vi "JoystickControls.vi"() -> (3 "input cluster":T1)   [LabVIEW 2015]
uses:
  Controls.ctl
  References/Refnums.vi
  <vilib>/Rock Robotics/WPI/Utilities/WPI_GetSetVariantRefNum.vi
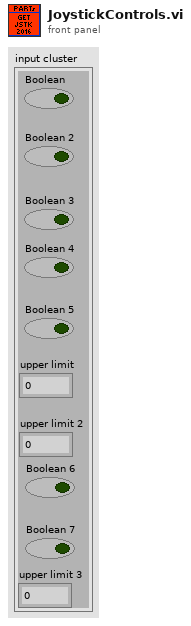
[diagram p1: front panel]
types:
  T1 = typedef "Controls.ctl" = cluster{"Boolean":bool, "Boolean 2":bool, "Boolean 3":bool, "Boolean 4":bool, "Boolean 5":bool, "upper limit":dbl, "upper limit 2":dbl, "Boolean 6":bool, "Boolean 7":bool, "upper limit 3":dbl}
  T2 = typedef "WPI_JoystickDevRef.ctl" = cluster{"Device":T3}
  T3 = typedef "WPI_JoystickDeviceEnum.ctl" = enum16{"USB 0", "USB 1", "USB 2", "USB 3", "USB 4", "USB 5"}
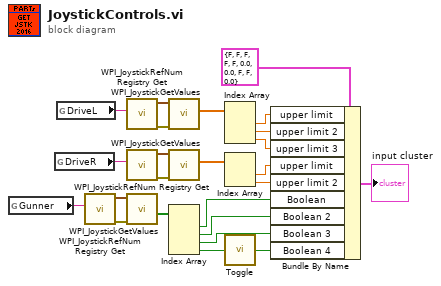
[diagram p0: block diagram]
diagram:
  n1 = global read "Refnums.vi" "Gunner"() -> (w23:string)
  n2 = global read "Refnums.vi" "DriveR"() -> (w8:string)
  n3 = global read "Refnums.vi" "DriveL"() -> (w22:string)
  n4 = call <vilib>:"WPI_JoystickRefNum Registry Get.vi"("refnum name"=w23) -> ("error out"=w18:errorcluster, "JoystickDevRef"=w19:T2)  [unwired: 9 in]
  n5 = call <vilib>:"WPI_JoystickRefNum Registry Get.vi"("refnum name"=w22) -> ("error out"=w21:errorcluster, "JoystickDevRef"=w20:T2)  [unwired: 9 in]
  n6 = call <vilib>:"WPI_JoystickRefNum Registry Get.vi"("refnum name"=w8) -> ("error out"=w9:errorcluster, "JoystickDevRef"=w10:T2)  [unwired: 9 in]
  n7 = call <vilib>:"WPI_JoystickGetValues.vi"("error in (no error)"=w18, "JoystickDevRef"=w19) -> ("Buttons"=w24:bool[])  [unwired: 5 in, 4 out]
  n8 = call <vilib>:"WPI_JoystickGetValues.vi"("error in (no error)"=w21, "JoystickDevRef"=w20) -> ("Axes"=w15:dbl[])  [unwired: 5 in, 4 out]
  n9 = call <vilib>:"WPI_JoystickGetValues.vi"("error in (no error)"=w9, "JoystickDevRef"=w10) -> ("Axes"=w11:dbl[])  [unwired: 5 in, 4 out]
  n10 = Index Array(array=w24) -> (element #1=w5:bool, element #2=w4:bool, element #3=w3:bool, element #4=w2:bool)  [unwired: 4 in]
  n11 = Index Array(array=w15) -> (element #1=w14:dbl, element #2=w13:dbl, element #3=w12:dbl)  [unwired: 3 in]
  n12 = Index Array(array=w11) -> (element #1=w7:dbl, element #2=w6:dbl)  [unwired: 2 in]
  n13 = call "Toggle.vi"("Input"=w2) -> ("Output"=w1:bool)  [unwired: 4 in]
  n14 = Bundle By Name(cluster=T1 {"Boolean"=FALSE, "Boolean 2"=FALSE, "Boolean 3"=FALSE, "Boolean 4"=FALSE, "Boolean 5"=FALSE, "upper limit"=0.0, "upper limit 2"=0.0, "Boolean 6"=FALSE, "Boolean 7"=FALSE, "upper limit 3"=0.0} ("input cluster"), "upper limit"=w14, "upper limit 2"=w13, "upper limit 3"=w12, "upper limit"=w7, "upper limit 2"=w6, "Boolean"=w5, "Boolean 2"=w4, "Boolean 3"=w3, "Boolean 4"=w1) -> (→"input cluster":T1)
